vi "Vision Express Tester.vi"   [LabVIEW 2016]
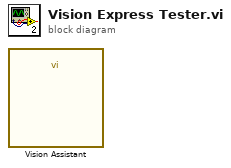
[diagram p0: block diagram]
diagram:
  n1 = call "Vision Assistant"() -> ()  [unwired: 26 in, 2 out]
